vi "Unpacking Data.vi"() -> ()   [LabVIEW 2019]
uses:
  <vilib>/Utility/file.llb/Read Delimited Spreadsheet (DBL).vi
  <vilib>/express/express analysis/Spectral/Block/exnSpectralBlock spectral measurements peak poly.vi
  <vilib>/express/express analysis/Spectral/Block/exnSpectralBlock spectral measurements peak WFM.vi
  <vilib>/express/express analysis/Spectral/XNode/ExpressSpectralMeasurementsBlockNode.xnode
panel:
  out "Waveform Graph 2":cluster{"f0":dbl, "df":dbl, "magnitude":dbl[]}(graph)
  out "Waveform Graph":waveform(dbl)(graph)
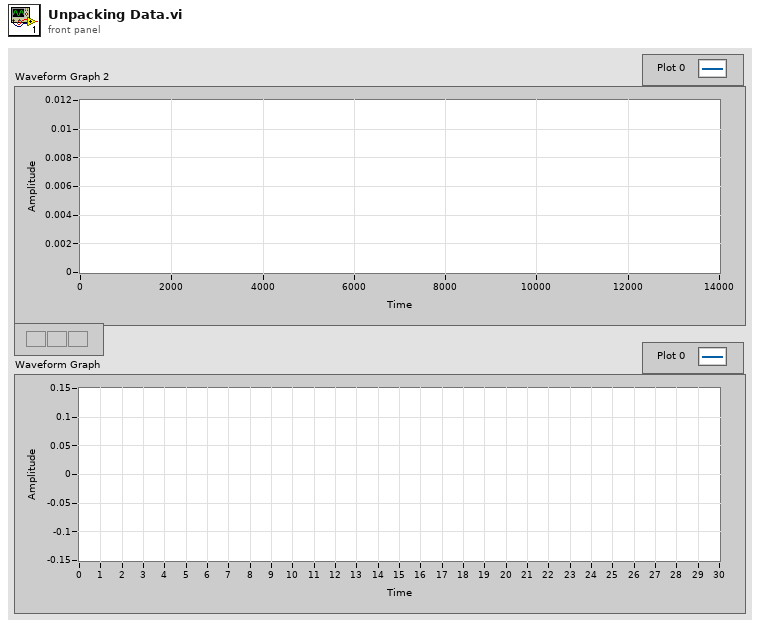
[diagram p1: front panel]
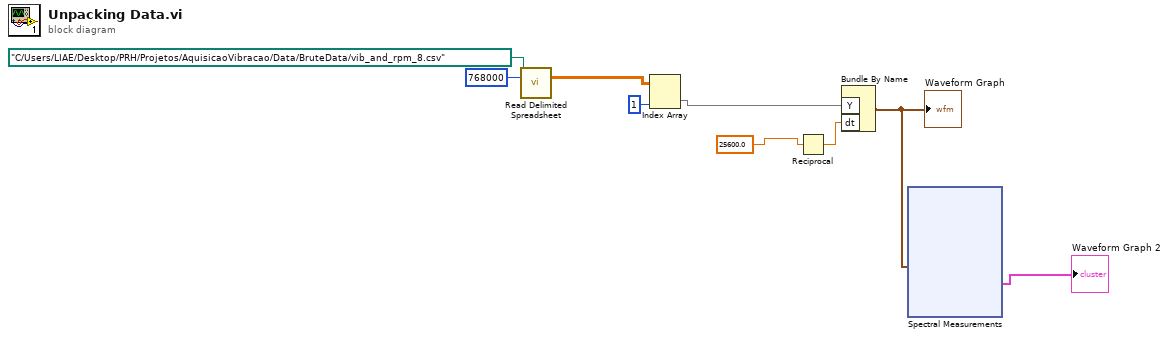
[diagram p0: block diagram]
diagram:
  n1 = call-poly <vilib>:"Read Delimited Spreadsheet.vi"("file path (dialog if empty)"=path "C:/Users/LIAE/Desktop/PRH/Projetos/AquisicaoVibracao/Data/BruteData/vib_and_rpm_8.csv", "number of rows (all:-1)"=768000) -> ("all rows"=w7:dbl[][])  [unwired: 8 in, 5 out]
  n2 = Index Array(array=w7, index (col)=1 ("disabled index (col)")) -> (element=w3:dbl[])  [unwired: 1 in]
  n3 = Reciprocal(x=25600.0 ("dt")) -> (1/x=w4:dbl)
  n4 = Bundle By Name("Y"=w3, "dt"=w4) -> (w2:waveform(dbl))  [unwired: 1 in]
  "Waveform Graph" <- w2
  n5 = xnode "Spectral Measurements"("Signals"=w2) -> ("FFT - (Peak)"=→"Waveform Graph 2":cluster{"f0":dbl, "df":dbl, "magnitude":dbl[]})  [unwired: 1 in, 2 out]
